vi "Write Current champion_.vi"(8 "error in (no error)":errorcluster, 10 "Current champion?":bool, 11 "WWF Wrestler in":refnum<class "WWE Wrestler.lvclass">) -> (0 "error out":errorcluster, 3 "WWF Wrestler out":refnum<class "WWE Wrestler.lvclass">)   [LabVIEW 2019, in "WWE Wrestler.lvclass"]
uses:
  WWE Wrestler.lvclass
  WWE Wrestler.lvclass/WWE Wrestler.ctl
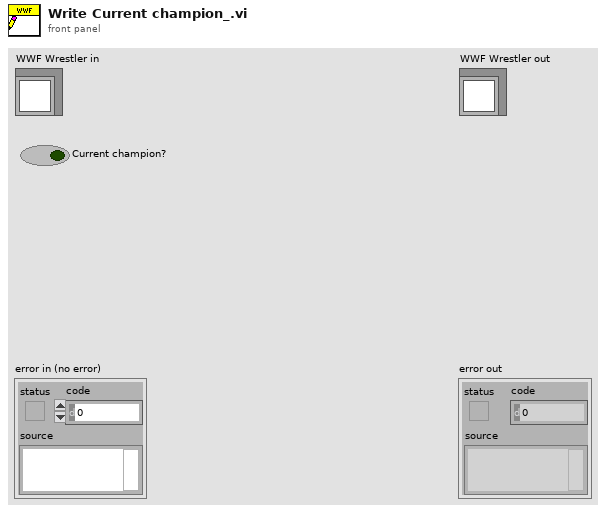
[diagram p1: front panel]
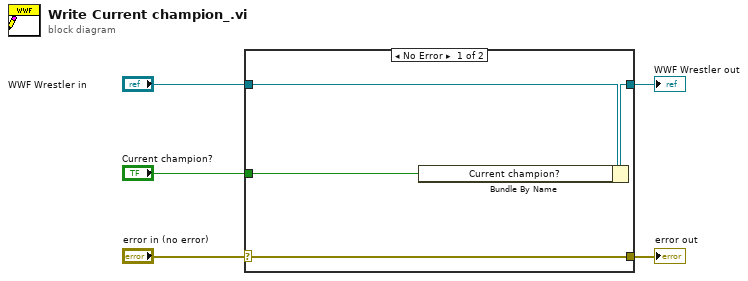
[diagram p0: block diagram]
diagram:
  n1 = case shown="No Error" "error in (no error)" {
    selector: "error in (no error)" -> [w9 w10]
    tunnel: [w9 w10] -> w4
    tunnel: [w7 w11] -> w2
    tunnel: "WWF Wrestler in" -> [w8 w11]
    tunnel: "Current champion?" -> [w6 _]
    frame No Error {
      n2 = Bundle By Name(cluster=w8, "Current champion?"=w6) -> (w7:refnum<class "WWE Wrestler.lvclass">)
    }
    frame Error {
    }
  }
  "error out" <- w4
  "WWF Wrestler out" <- w2
